vi "Get Project Data.vi"(8 "error in":errorcluster, 10 "Target Selection":string, 11 "Project Selection":string) -> (0 "error out":errorcluster, 3 "Project Data":T1)   [LabVIEW 2020, in "ConstantErrorsMaker.lvlib"]
uses:
  ConstantErrorsMaker.lvlib
  Project Data--cluster.ctl
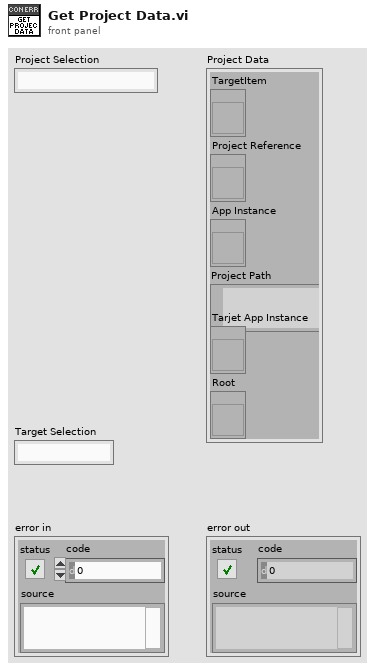
[diagram p1: front panel]
types:
  T1 = typedef "ConstantErrorsMaker.lvlib/Project Data--cluster.ctl" = cluster{"TargetItem":refnum<vi>, "Project Reference":refnum<vi>, "App Instance":refnum<vi>, "Project Path":path, "Tarjet App Instance":refnum<vi>, "Root":refnum<vi>}
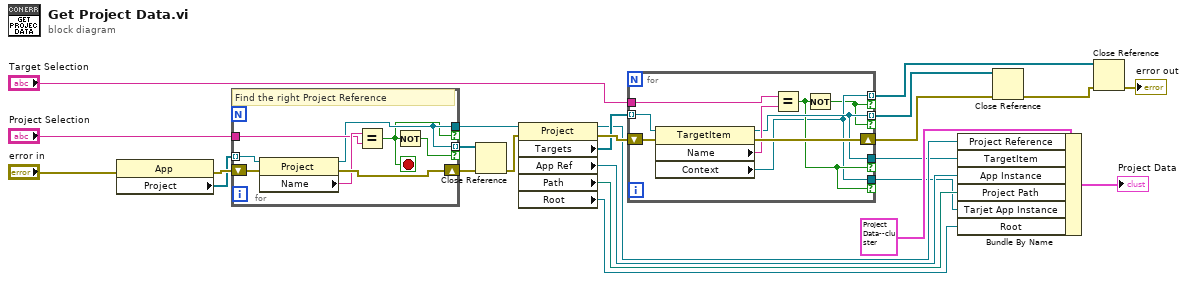
[diagram p0: block diagram]
diagram:
  n1 = property class="App"(error in="error in") -> (error out=w22:errorcluster, "Project"=w15:refnum<vi>[])  [unwired: 1 in, 1 out]
  n2 = for {
    tunnel: [w28] -> w10 if=w27
    tunnel: "Project Selection" -> [w29]
    tunnel: [w28] -> w14 mode=indexing if=w26
    tunnel: w15 -> [w25] mode=indexing
    shift-right: [w32] -> w23
    shift-left: w22 -> [w31]
    stop <- w27 stop-if-true
    # "Find the right Project Reference"
    n3 = property class="Project"(reference=w25, error in=w31) -> (reference out=w28:refnum<vi>, error out=w32:errorcluster, "Name"=w30:string)
    n4 = Equal?(x=w30, y=w29) -> (x = y?=w27:bool)
    n5 = Not(x=w27) -> (.not. x?=w26:bool)
  }
  n6 = Close Reference(reference=w14, error in (no error)=w23) -> (error out=w18:errorcluster)
  n7 = property class="Project"(reference=w10, error in=w18) -> (reference out=w7:refnum<vi>, error out=w20:errorcluster, "Targets"=w12:refnum<vi>[], "App Ref"=w5:refnum<vi>, "Path"=w4:path, "Root"=w1:refnum<vi>)
  n8 = for {
    tunnel: w12 -> [w39] mode=indexing
    tunnel: [w37] -> w6 if=w36
    tunnel: [w37] -> w13 mode=indexing if=w34
    shift-right: [w40] -> w19
    shift-left: w20 -> [w41]
    tunnel: [w35] -> w2 if=w36
    tunnel: [w35] -> w11 mode=indexing if=w34
    tunnel: "Target Selection" -> [w33]
    n9 = property class="TargetItem"(reference=w39, error in=w41) -> (reference out=w37:refnum<vi>, error out=w40:errorcluster, "Name"=w38:string, "Context"=w35:refnum<vi>)
    n10 = Equal?(x=w33, y=w38) -> (x = y?=w36:bool)
    n11 = Not(x=w36) -> (.not. x?=w34:bool)
  }
  n12 = Bundle By Name(cluster=T1 {"TargetItem"=refnum, "Project Reference"=refnum, "App Instance"=refnum, "Project Path"=path "", "Tarjet App Instance"=refnum, "Root"=refnum} ("Project Data"), "Project Reference"=w7, "TargetItem"=w6, "App Instance"=w5, "Project Path"=w4, "Tarjet App Instance"=w2, "Root"=w1) -> (→"Project Data":T1)
  n13 = Close Reference(reference=w13, error in (no error)=w19) -> (error out=w21:errorcluster)
  n14 = Close Reference(reference=w11, error in (no error)=w21) -> (error out=→"error out":errorcluster)
